vi "Look Up Indexes.vi"(5 "outgoing channels":refnum<class "TBM channel.lvclass">[](array[class]), 7 "incoming channels":refnum<class "TBM channel.lvclass">[](array[class]), 8 "error in":errorcluster, 9 "Incoming Single Point Configuraiton in":T6, 10 "Outgoing Cyclic Configuration in":T1 {"Outgoing Cyclic Frame"."Transmit Propreties"."Transmit Time" format="%#_p"}, 11 "data allocations in":T8) -> (0 "error out":errorcluster, 1 "Incoming Single Point Configuraiton out":T6, 2 "Outgoing Cyclic Configuration out":T1 {"Outgoing Cyclic Frame"."Transmit Propreties"."Transmit Time" format="%#_p"}, 3 "data allocations out":T8)   [LabVIEW 2013, in "J1939.lvlib"]
uses:
  J1939.lvlib
  <vilib>/NI/Tag Bus Module Framework/channel/data tables.ctl
  <vilib>/NI/Tag Bus/dictionary/data dictionary.lvclass
  <vilib>/NI/Tag Bus/dictionary table pair.ctl
  <vilib>/NI/Tag Bus/table/data table.ctl
  CD/CD Incoming Single Point Configuration.ctl
  CD/CD Incoming Single Point Frame Pairs.ctl
  module/configuration/Signal Mapping.ctl
  <vilib>/NI/Tag Bus/tag/Data Type.ctl
  CD/CD Outgoing Cyclic Configuration.ctl
  CD/CD Outgoing Cyclic Frame Pairs.ctl
  API Types/XNET Frame Event Properties.ctl
  <vilib>/NI/Tag Bus Module Framework/channel/TBM channel.lvclass
  <vilib>/NI/Tag Bus/tag/tag descriptor.lvclass/tag descriptor.ctl
  <vilib>/NI/Tag Bus/tag/read tag name.vi
  <vilib>/NI/Tag Bus/tag/read data type.vi
  <vilib>/NI/Tag Bus/dictionary/locate tag.vi
  <vilib>/NI/Tag Bus/table/data table.lvlib
  <vilib>/NI/Tag Bus/tag bus.lvlib
  <vilib>/NI/Tag Bus/tag/tag descriptor.lvclass
  module/configuration/J1939 configuration.lvclass
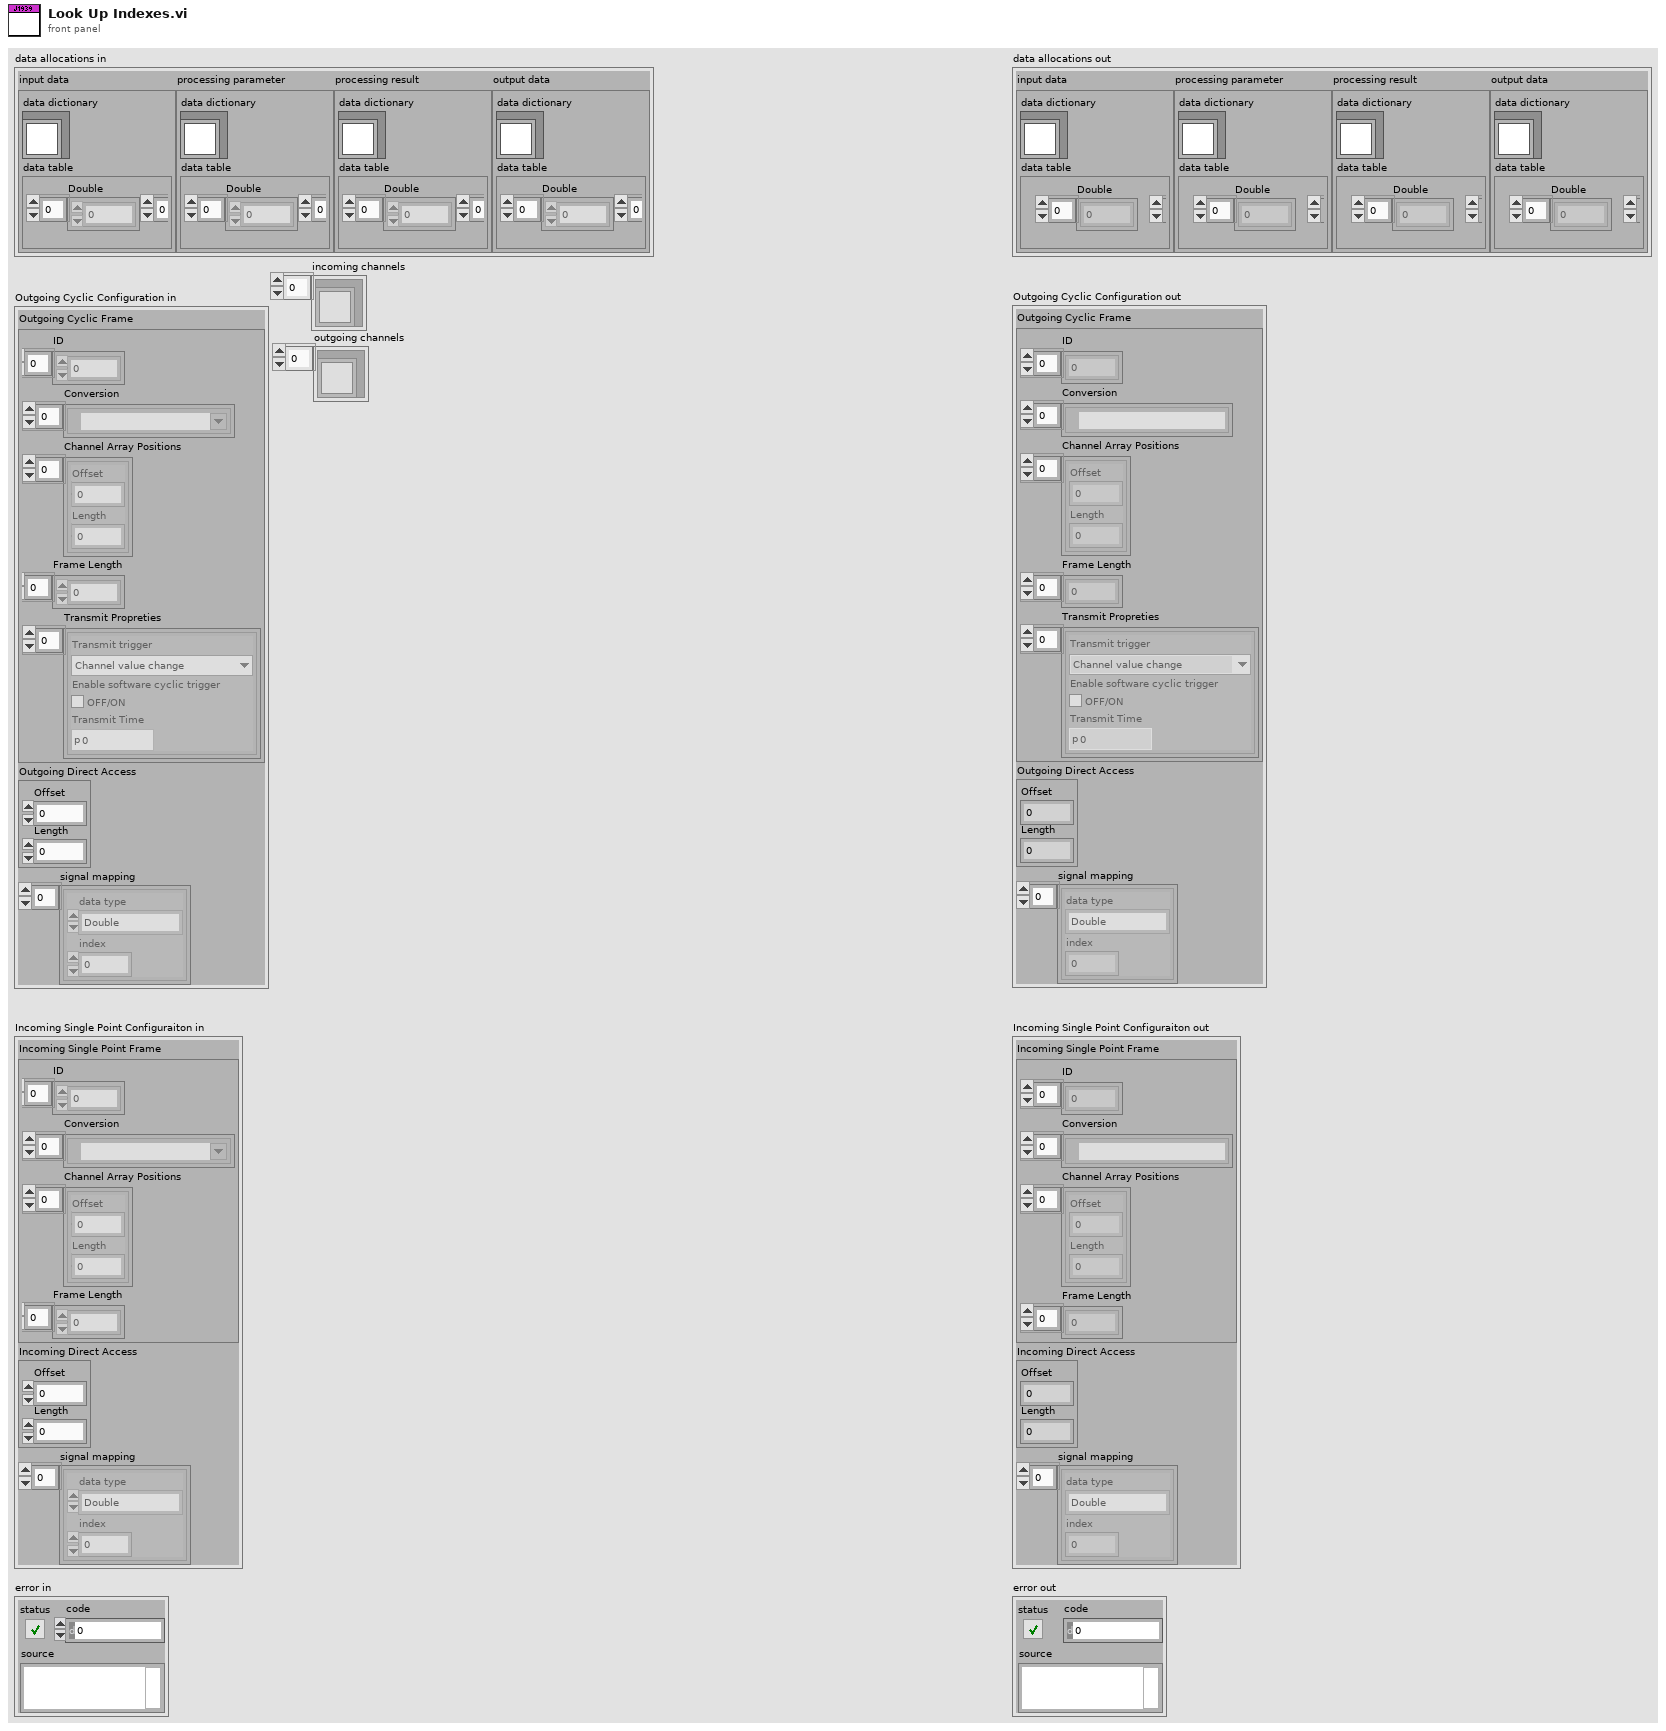
[diagram p1: front panel]
types:
  T1 = typedef "J1939.lvlib/CD Outgoing Cyclic Configuration.ctl" = cluster{"Outgoing Cyclic Frame":T2, "Outgoing Direct Access":cluster{"Offset":u32, "Length":u32}, "signal mapping":T4[]}
  T2 = typedef "J1939.lvlib/CD Outgoing Cyclic Frame Pairs.ctl" = cluster{"ID":u32[], "Conversion":refnum<k21>[], "Channel Array Positions":cluster{"Offset":u32, "Length":u32}[], "Frame Length":u32[], "Transmit Propreties":T3[]}
  T3 = typedef "J1939.lvlib/XNET Frame Event Properties.ctl" = cluster{"Transmit trigger":enum16{"Channel value change"}, "Enable software cyclic trigger":bool, "Transmit Time":dbl}
  T4 = typedef "J1939 configuration.lvclass/Signal Mapping.ctl" = cluster{"data type":T5, "index":i32}
  T5 = typedef "tag bus.lvlib/tag descriptor.lvclass/Data Type.ctl" = enum16{"Double", "Single", "I64", "I32", "I16", "I8", "U64", "U32", "U16", "U8", "Boolean", "String", "Array of Double", "Array of Single", "Array of I64", "Array of I32", "Array of I16", "Array of I8", "Array of U64", "Array of U32", "Array of U16", "Array of U8", "Array of Boolean", "Array of String"}
  T6 = typedef "J1939.lvlib/CD Incoming Single Point Configuration.ctl" = cluster{"Incoming Single Point Frame":T7, "Incoming Direct Access":cluster{"Offset":u32, "Length":u32}, "signal mapping":T4[]}
  T7 = typedef "J1939.lvlib/CD Incoming Single Point Frame Pairs.ctl" = cluster{"ID":u32[], "Conversion":refnum<k21>[], "Channel Array Positions":cluster{"Offset":u32, "Length":u32}[], "Frame Length":u32[]}
  T8 = typedef "TBM channel.lvclass/data tables.ctl" = cluster{"input data":T9, "processing parameter":T9, "processing result":T9, "output data":T9}
  T9 = typedef "tag bus.lvlib/dictionary table pair.ctl" = cluster{"data dictionary":refnum<class "data dictionary.lvclass">, "data table":T10}
  T10 = typedef "tag bus.lvlib/data table.lvlib/data table.ctl" = cluster{"Double":dbl[], "Single":sgl[], "I64":i64[], "I32":i32[], "I16":i16[], "I8":i8[], "U64":u64[], "U32":u32[], "U16":u16[], "U8":u8[], "Boolean":bool[], "String":string[], "Array of Double":cluster{"DBL Array":dbl[]}[], "Array of Single":cluster{"SGL Array":sgl[]}[], "Array of I64":cluster{"I64 Array":i64[]}[], "Array of I32":cluster{"I32 Array":i32[]}[], "Array of I16":cluster{"I16 Array":i16[]}[], "Array of I8":cluster{"I8 Array":i8[]}[], "Array of U64":cluster{"U64 Array":u64[]}[], "Array of U32":cluster{"U32 Array":u32[]}[], "Array of U16":cluster{"U16 Array":u16[]}[], "Array of U8":cluster{"U8 Array":u8[]}[], "Array of Boolean":cluster{"Boolean Array":bool[]}[], "Array of String":cluster{"String Array":string[]}[]}
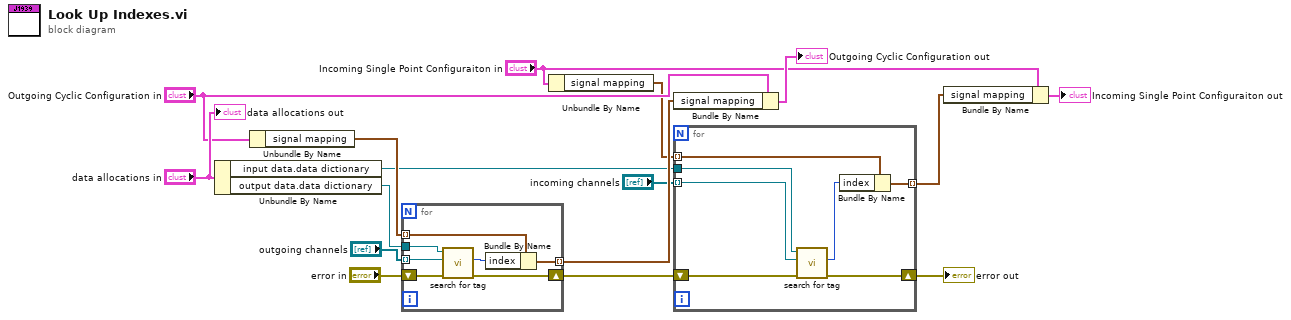
[diagram p0: block diagram]
diagram:
  n1 = Unbundle By Name("data allocations in") -> ("input data.data dictionary"=w6:refnum<class "data dictionary.lvclass">, "output data.data dictionary"=w14:refnum<class "data dictionary.lvclass">)
  n2 = Unbundle By Name("Outgoing Cyclic Configuration in") -> ("signal mapping"=w12:T4[])
  n3 = for {
    shift-right: [w21] -> w7
    shift-left: "error in" -> [w23]
    tunnel: w14 -> [w22]
    tunnel: w12 -> [w20] mode=indexing
    tunnel: [w18] -> w11 mode=indexing
    tunnel: "outgoing channels" -> [w17] mode=indexing
    n4 = call <vilib>:"search for tag.vi"("error in"=w23, "system tag"=w17, "data dictionary in"=w22) -> ("error out"=w21:errorcluster, "index"=w19:i32)  [unwired: 6 in, 1 out]
    n5 = Bundle By Name(cluster=w20, "index"=w19) -> (w18:T4)
  }
  n6 = Unbundle By Name("Incoming Single Point Configuraiton in") -> ("signal mapping"=w8:T4[])
  n7 = Bundle By Name(cluster="Outgoing Cyclic Configuration in", "signal mapping"=w11) -> (→"Outgoing Cyclic Configuration out":T1)
  n8 = for {
    shift-right: [w28] -> w5
    shift-left: w7 -> [w30]
    tunnel: w6 -> [w29]
    tunnel: w8 -> [w27] mode=indexing
    tunnel: [w25] -> w9 mode=indexing
    tunnel: "incoming channels" -> [w24] mode=indexing
    n9 = call <vilib>:"search for tag.vi"("error in"=w30, "system tag"=w24, "data dictionary in"=w29) -> ("error out"=w28:errorcluster, "index"=w26:i32)  [unwired: 6 in, 1 out]
    n10 = Bundle By Name(cluster=w27, "index"=w26) -> (w25:T4)
  }
  "error out" <- w5
  n11 = Bundle By Name(cluster="Incoming Single Point Configuraiton in", "signal mapping"=w9) -> (→"Incoming Single Point Configuraiton out":T6)
  "data allocations out" <- "data allocations in"
